vi "Get API.vi"(8 "error in (no error)":errorcluster, 11 "Service in":refnum<class "Service.lvclass">) -> (0 "error out":errorcluster, 2 "API":string[](array[string]), 3 "Service out":refnum<class "Service.lvclass">)   [LabVIEW 2024, in "Ramses Framework.lvlib" / "Service.lvclass"]
uses:
  Service.lvclass
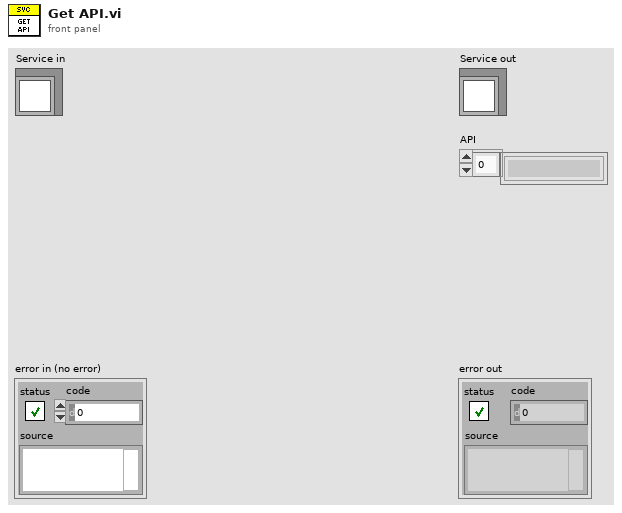
[diagram p1: front panel]
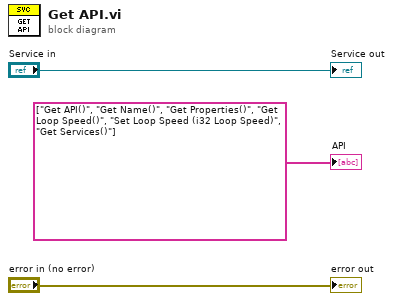
[diagram p0: block diagram]
diagram:
  "error out" <- "error in (no error)"
  "Service out" <- "Service in"
  "API" <- string[] ["Get API()", "Get Name()", "Get Properties()", "Get Loop Speed()", "Set Loop Speed (i32 Loop Speed)", "Get Services()"]
